vi "FreqsComponentesProximeter.vi"(2 "Tipo_ParamsProximeter":T1) -> (15 "AmplitComponentes":dbl[](array[numeric]), 16 "FreqsComponentes":dbl[](array[numeric]))   [LabVIEW 2017]
uses:
  Typedefs/Tipo_ParamsProximeter.ctl
  Typedefs/Tipo_ComponentesProximeter.ctl
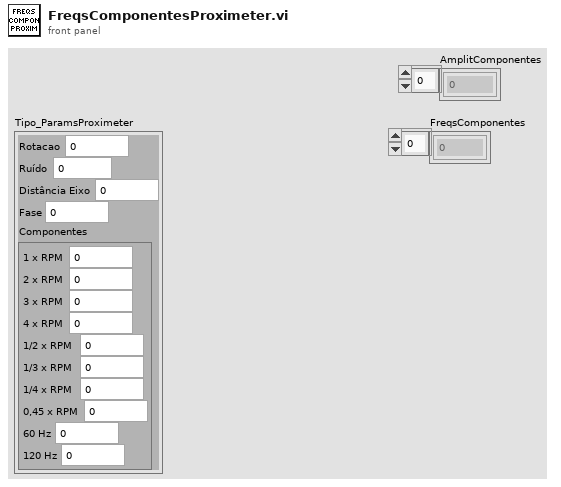
[diagram p1: front panel]
types:
  T1 = typedef "Tipo_ParamsProximeter.ctl" = cluster{"Rotacao":dbl, "Ruído":dbl, "Distância Eixo":dbl, "Fase":dbl, "Componentes":T2}
  T2 = typedef "Tipo_ComponentesProximeter.ctl" = cluster{"1xRPM":dbl, "2xRPM":dbl, "3xRPM":dbl, "4xRPM":dbl, "1/2xRPM":dbl, "1/3xRPM":dbl, "1/4xRPM":dbl, "0,45xRPM":dbl, "60Hz":dbl, "120Hz":dbl}
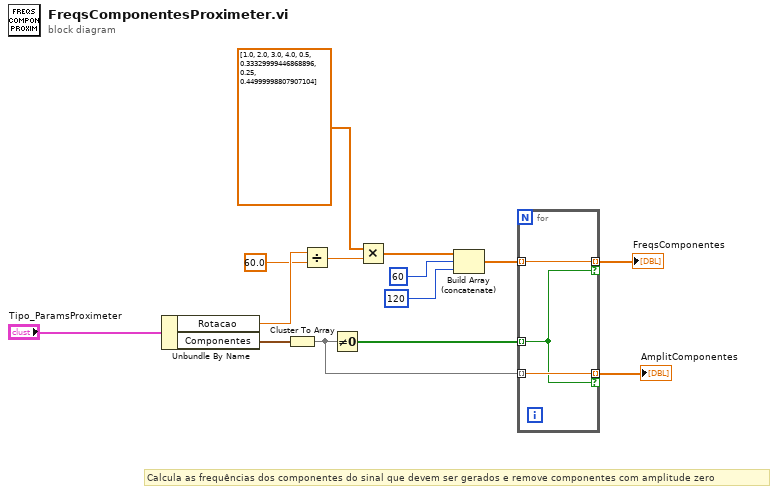
[diagram p0: block diagram]
diagram:
  # "Calcula as frequências dos componentes do sinal que devem ser gerados e remove componentes com amplitude zero"
  n1 = Unbundle By Name("Tipo_ParamsProximeter") -> ("Rotacao"=w12:dbl, "Componentes"=w13:T2)
  n2 = Cluster To Array(cluster=w13) -> (array=w2:dbl[])
  n3 = Divide(x=w12, y=60.0) -> (x/y=w10:dbl)
  n4 = Not Equal To 0?(x=w2) -> (x != 0?=w4:bool[])
  n5 = Multiply(x=sgl[] [1.0, 2.0, 3.0, 4.0, 0.5, 0.3333, 0.25, 0.45], y=w10) -> (x*y=w8:dbl[])
  n6 = Build Array (concatenate)(w8, 60, 120) -> (w5:dbl[])
  n7 = for {
    tunnel: w5 -> [w17] mode=indexing
    tunnel: w4 -> [w15] mode=indexing
    tunnel: [w17] -> w3 mode=indexing if=w15
    tunnel: w2 -> [w16] mode=indexing
    tunnel: [w16] -> w1 mode=indexing if=w15
  }
  "FreqsComponentes" <- w3
  "AmplitComponentes" <- w1
